vi "工况数据接口全局.vi"() -> ()   [LabVIEW 2022 SP3]
uses:
  <vilib>/ActorFramework/Message Enqueuer/Message Enqueuer.lvclass
panel:
  out "Actor's Enqueuer":refnum<class "Message Enqueuer.lvclass"> caption="操作者待入队列"
  out "sync":bool
  in  "data":T1={"time"="2021-05-08 14-02-02", "data"={"ups"={"ups"={"input_voltage"=0.0, "input_frequency"=0.0, "output_voltage"=0.0, "output_current"=0.0, "output_frequency"=0.0, "output_active_power"=0.0, "output_apparent_power"=0.0, "load_rate"=0.0, "cabinet_temperature"=0.0, "battery_voltage"=0.0, "remaining_battery_capacity"=0.0, "power_on_status"="", "power_supply_mode"="", "fault"=FALSE, "battery_low_voltage"=FALSE, "mains_supply_abnormality"=FALSE}, "启用"=FALSE}, "air_conditioner"={"air_conditioner"={"cabinet_temperature"=0.0, "air_supply_temperature"=0.0, "voltage"=0.0, "current"=0.0, "compressor_status"="", "Internal_fan_status"="", "external_fan_status"="", "heating_state"="", "refrigeration_state"=FALSE, "high_temperature_alarm"=FALSE, "low_temperature_alarm"=FALSE, "heater_fault"=FALSE, "temperature_sensor_fault"=FALSE, "high_voltage_alarm"=FALSE, "low_voltage_alarm"=FALSE, "refrigeration_start_point"=0.0, "refrigeration_sensitive_point"=0.0, "heating_start_point"=0.0, "heating_sensitive_point"=0.0, "high_temperature_alarm_point"=0.0, "low_temperature_alarm_point"=0.0}, "启用"=FALSE}, "smoke_sensor"={"smoke_sensor"={"trigger_alarm"=FALSE}, "启用"=FALSE}, "water_immersion_sensor"={"water_immersion_sensor"={"trigger_alarm"=FALSE}, "启用"=FALSE}, "temperature_and_humidity_sensor"={"temperature_and_humidity_sensor"={"current_temperature"=0.0, "current_humidity"=0.0, "room_temperature_alarm"=FALSE, "humidity_alarm"=FALSE}, "启用"=FALSE}, "gps"={"gps"={"current_longitude"=0.0, "current_latitude"=0.0, "launch_longitude"=0.0, "launch_latitude"=0.0, "shift_alarm"=FALSE}, "启用"=FALSE}, "solar_controller"={"solar_controller"={"array_voltage"=0.0, "array_current"=0.0, "generating_power"=0.0, "battery_voltage"=0.0, "battery_current"=0.0, "ceiling_voltage"=0.0, "minimum_voltage"=0.0, "battery_temperature"=0.0, "remaining_battery_capacity"=0.0, "load_voltage"=0.0, "load_current"=0.0, "load_power"=0.0, "equipment_temperature"=0.0, "accumulated_electricity_consumption_of_the_day"=0.0, "accumulated_electricity_consumption_of_the_current_month"=0.0, "accumulated_electricity_consumption_in_the_current_year"=0.0, "total_accumulated_power_consumption"=0.0, "accumulated_charging_capacity_of_the_day"=0.0, "accumulated_charging_amount_of_the_current_month"=0.0, "accumulated_charging_capacity_of_the_current_year"=0.0, "total_cumulative_charge"=0.0}, "启用"=FALSE}, "solar_controller_2"={"solar_controller_2"={"array_voltage"=0.0, "array_current"=0.0, "generating_power"=0.0, "battery_voltage"=0.0, "battery_current"=0.0, "ceiling_voltage"=0.0, "minimum_voltage"=0.0, "battery_temperature"=0.0, "remaining_battery_capacity"=0.0, "load_voltage"=0.0, "load_current"=0.0, "load_power"=0.0, "equipment_temperature"=0.0, "accumulated_electricity_consumption_of_the_day"=0.0, "accumulated_electricity_consumption_of_the_current_month"=0.0, "accumulated_electricity_consumption_in_the_current_year"=0.0, "total_accumulated_power_consumption"=0.0, "accumulated_charging_capacity_of_the_day"=0.0, "accumulated_charging_amount_of_the_current_month"=0.0, "accumulated_charging_capacity_of_the_current_year"=0.0, "total_cumulative_charge"=0.0}, "启用"=FALSE}, "NH3"={"NH3"={"F0"=0.0, "F1"=0.0, "syringe_temperature"=0.0, "alarm_step"=0.0, "X0"=0.0}, "启用"=FALSE}, "TP"={"TP"={"F0"=0.0, "F1"=0.0, "F2"=0.0, "F3"=0.0, "digestion_temperature"=0.0, "constant_temperature"=0.0, "syringe_temperature"=0.0, "alarm_step"=0.0, "X0"=0.0}, "启用"=FALSE}, "TN"={"TN"={"F0"=0.0, "F1"=0.0, "F2"=0.0, "F3"=0.0, "F4"=0.0, "F5"=0.0, "F6"=0.0, "F7"=0.0, "digestion_temperature"=0.0, "constant_temperature"=0.0, "syringe_temperature"=0.0, "alarm_step"=0.0, "X0"=0.0}, "启用"=FALSE}, "CODMn"={"CODMn"={"temperature_curve"=[], "titration_curve"=[], "F0"=0.0, "F1"=0.0, "F2"=0.0, "F3"=0.0, "F4"=0.0, "F5"=0.0, "A"=0.0, "B"=0.0, "K"=0.0}, "启用"=FALSE}, "CODCr"={"CODCr"={"temperature_curve"=[], "F0"=0.0, "F1"=0.0, "reagent_sensor"=0.0}, "启用"=FALSE}}} {"data"."air_conditioner"."air_conditioner"."current" format="%#.2g"}
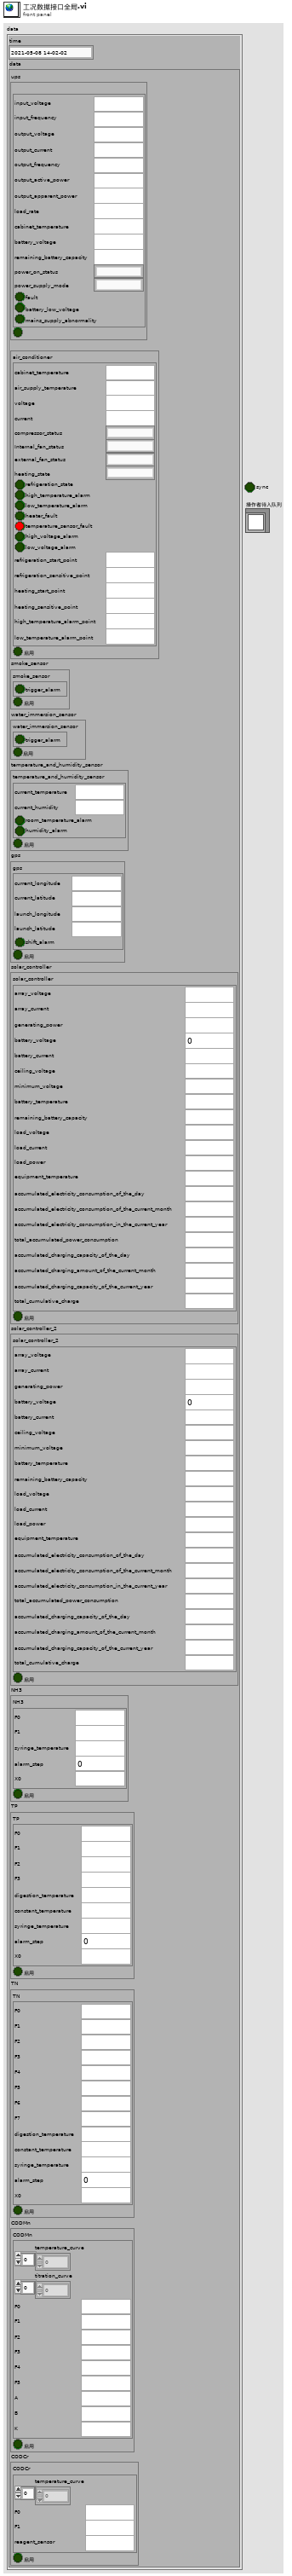
[diagram p1: front panel]
types:
  T1 = typedef "工况数据.ctl" = cluster{"time":string, "data":cluster{"ups":cluster{"ups":cluster{"input_voltage":ext, "input_frequency":ext, "output_voltage":ext, "output_current":ext, "output_frequency":ext, "output_active_power":ext, "output_apparent_power":ext, "load_rate":ext, "cabinet_temperature":ext, "battery_voltage":ext, "remaining_battery_capacity":ext, "power_on_status":string, "power_supply_mode":string, "fault":bool, "battery_low_voltage":bool, "mains_supply_abnormality":bool}, "启用":bool}, "air_conditioner":cluster{"air_conditioner":cluster{"cabinet_temperature":ext, "air_supply_temperature":ext, "voltage":ext, "current":ext, "compressor_status":string, "Internal_fan_status":string, "external_fan_status":string, "heating_state":string, "refrigeration_state":bool, "high_temperature_alarm":bool, "low_temperature_alarm":bool, "heater_fault":bool, "temperature_sensor_fault":bool, "high_voltage_alarm":bool, "low_voltage_alarm":bool, "refrigeration_start_point":ext, "refrigeration_sensitive_point":ext, "heating_start_point":ext, "heating_sensitive_point":ext, "high_temperature_alarm_point":ext, "low_temperature_alarm_point":ext}, "启用":bool}, "smoke_sensor":cluster{"smoke_sensor":cluster{"trigger_alarm":bool}, "启用":bool}, "water_immersion_sensor":cluster{"water_immersion_sensor":cluster{"trigger_alarm":bool}, "启用":bool}, "temperature_and_humidity_sensor":cluster{"temperature_and_humidity_sensor":cluster{"current_temperature":ext, "current_humidity":ext, "room_temperature_alarm":bool, "humidity_alarm":bool}, "启用":bool}, "gps":cluster{"gps":cluster{"current_longitude":ext, "current_latitude":ext, "launch_longitude":ext, "launch_latitude":ext, "shift_alarm":bool}, "启用":bool}, "solar_controller":cluster{"solar_controller":cluster{"array_voltage":ext, "array_current":ext, "generating_power":ext, "battery_voltage":dbl, "battery_current":ext, "ceiling_voltage":ext, "minimum_voltage":ext, "battery_temperature":ext, "remaining_battery_capacity":ext, "load_voltage":ext, "load_current":ext, "load_power":ext, "equipment_temperature":ext, "accumulated_electricity_consumption_of_the_day":ext, "accumulated_electricity_consumption_of_the_current_month":ext, "accumulated_electricity_consumption_in_the_current_year":ext, "total_accumulated_power_consumption":ext, "accumulated_charging_capacity_of_the_day":ext, "accumulated_charging_amount_of_the_current_month":ext, "accumulated_charging_capacity_of_the_current_year":ext, "total_cumulative_charge":ext}, "启用":bool}, "solar_controller_2":cluster{"solar_controller_2":cluster{"array_voltage":ext, "array_current":ext, "generating_power":ext, "battery_voltage":dbl, "battery_current":ext, "ceiling_voltage":ext, "minimum_voltage":ext, "battery_temperature":ext, "remaining_battery_capacity":ext, "load_voltage":ext, "load_current":ext, "load_power":ext, "equipment_temperature":ext, "accumulated_electricity_consumption_of_the_day":ext, "accumulated_electricity_consumption_of_the_current_month":ext, "accumulated_electricity_consumption_in_the_current_year":ext, "total_accumulated_power_consumption":ext, "accumulated_charging_capacity_of_the_day":ext, "accumulated_charging_amount_of_the_current_month":ext, "accumulated_charging_capacity_of_the_current_year":ext, "total_cumulative_charge":ext}, "启用":bool}, "NH3":cluster{"NH3":cluster{"F0":ext, "F1":ext, "syringe_temperature":ext, "alarm_step":dbl, "X0":ext}, "启用":bool}, "TP":cluster{"TP":cluster{"F0":ext, "F1":ext, "F2":ext, "F3":ext, "digestion_temperature":ext, "constant_temperature":ext, "syringe_temperature":ext, "alarm_step":dbl, "X0":ext}, "启用":bool}, "TN":cluster{"TN":cluster{"F0":ext, "F1":ext, "F2":ext, "F3":ext, "F4":ext, "F5":ext, "F6":ext, "F7":ext, "digestion_temperature":ext, "constant_temperature":ext, "syringe_temperature":ext, "alarm_step":dbl, "X0":ext}, "启用":bool}, "CODMn":cluster{"CODMn":cluster{"temperature_curve":ext[], "titration_curve":ext[], "F0":ext, "F1":ext, "F2":ext, "F3":ext, "F4":ext, "F5":ext, "A":ext, "B":ext, "K":ext}, "启用":bool}, "CODCr":cluster{"CODCr":cluster{"temperature_curve":ext[], "F0":ext, "F1":ext, "reagent_sensor":ext}, "启用":bool}}}
diagram:
